vi "PAN_BuildDefModPath.vi"(9 "mod name":string, 10 "modpath":path) -> (2 "modapipath":path)   [LabVIEW 2016]
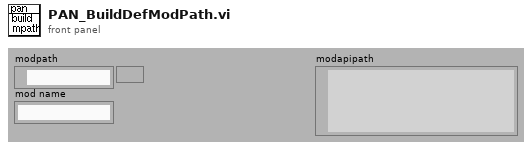
[diagram p1: front panel]
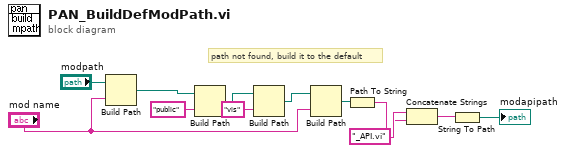
[diagram p0: block diagram]
diagram:
  # "path not found, build it to the default"
  n1 = Build Path(base path="modpath", name or relative path="mod name") -> (appended path=w12:path)
  n2 = Build Path(base path=w12, name or relative path="public") -> (appended path=w10:path)
  n3 = Build Path(base path=w10, name or relative path="vis") -> (appended path=w5:path)
  n4 = Build Path(base path=w5, name or relative path="mod name") -> (appended path=w4:path)
  n5 = Path To String(path=w4) -> (string=w8:string)
  n6 = Concatenate Strings(w8, "_API.vi" ("string")) -> (w6:string)
  n7 = String To Path(string=w6) -> (path=→"modapipath":path)
